vi "SeqRelease.vi"(8 "error in":errorcluster, 11 "Index":i32) -> (0 "error out":errorcluster, 4 "return":i32)   [LabVIEW 2019]
uses:
  [Global] Image.vi
  [Global] Image Overlay.vi
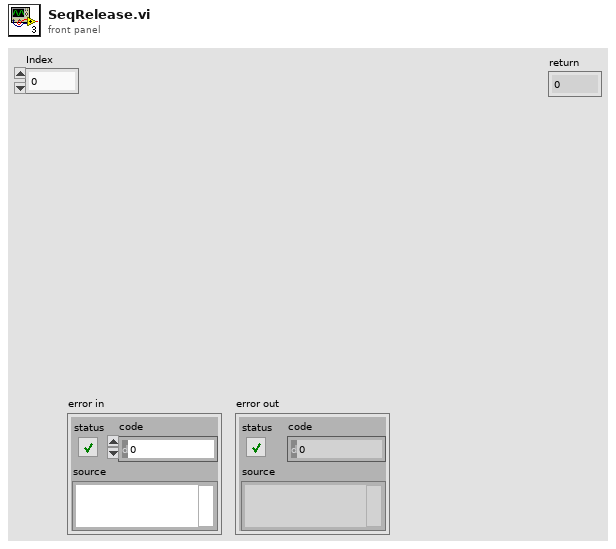
[diagram p1: front panel]
types:
  T1 = typedef "IMAQ Image.ctl" = refnum<image>
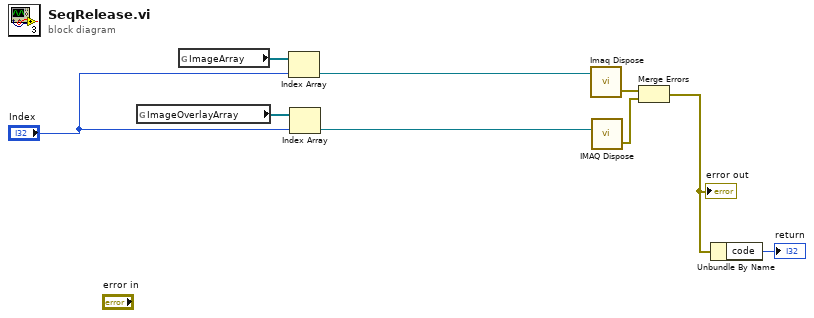
[diagram p0: block diagram]
diagram:
  n1 = global read "[Global] Image Overlay.vi" "ImageOverlayArray"() -> (w3:T1[])
  n2 = global read "[Global] Image.vi" "ImageArray"() -> (w5:T1[])
  n3 = Index Array(array=w5, index="Index") -> (element=w4:T1)
  n4 = Index Array(array=w3, index="Index") -> (element=w1:T1)
  n5 = call "Imaq Dispose"("Image"=w4) -> ("error out"=w8:errorcluster)  [unwired: 5 in]
  n6 = call "IMAQ Dispose"("Image"=w1) -> ("error out"=w7:errorcluster)  [unwired: 5 in]
  n7 = Merge Errors(w8, w7) -> (w6:errorcluster)
  "error out" <- w6
  n8 = Unbundle By Name(w6) -> ("code"=→"return":i32)
